vi "filterReadTimeout.vi"(8 "error in (no error)":errorcluster, 9 "matchChar":string, 10 "timeoutMs":u32=2000, 11 "filterPort":refnum<visa-resource-name>) -> (0 "error out":errorcluster, 2 "rxData":string, 3 "filterPortOut":refnum<visa-resource-name>)   [LabVIEW 2018]
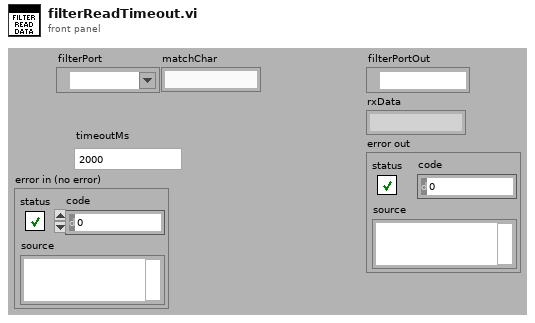
[diagram p1: front panel]
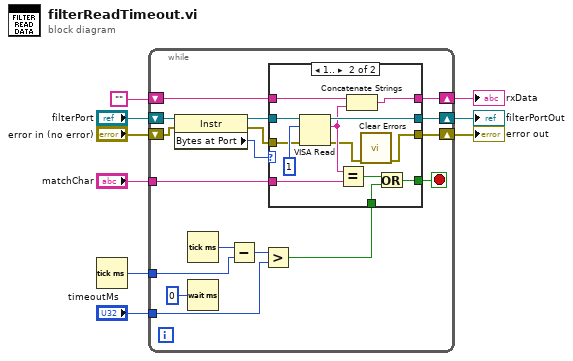
[diagram p0: block diagram]
diagram:
  n1 = Tick Count (ms)() -> (millisecond timer value=w8:u32)
  n2 = while {
    shift-left: "" -> [w25]
    shift-right: [w26] -> w4
    shift-right: [w23] -> w5
    shift-left: "filterPort" -> [w24]
    tunnel: w8 -> [w21]
    tunnel: "timeoutMs" -> [w18]
    shift-right: [w14] -> w2
    shift-left: "error in (no error)" -> [w15]
    tunnel: "matchChar" -> [w12]
    stop <- w11 stop-if-true
    n3 = property class="Instr"(reference=w24, error in=w15) -> (reference out=w17:refnum<visa-resource-name>, error out=w13:errorcluster, "Bytes at Port"=w16:u32)
    n4 = Tick Count (ms)() -> (millisecond timer value=w22:u32)
    n5 = Wait (ms)(milliseconds to wait=u32 0) -> ()  [unwired: 1 out]
    n6 = Subtract(x=w22, y=w21) -> (x-y=w20:u32)
    n7 = Greater?(x=w20, y=w18) -> (0:w10:bool)
    n8 = case shown="1.." w16 {
      tunnel: [w30 w43] -> w26
      tunnel: w25 -> [w30 w42]
      tunnel: [w29 w41] -> w23
      tunnel: w17 -> [w29 w39]
      tunnel: [w28 w31] -> w14
      tunnel: w13 -> [w28 w38]
      tunnel: w12 -> [_ w36]
      tunnel: [w27 w34] -> w11
      tunnel: w10 -> [w27 w33]
      frame 0, Default {
      }
      frame 1.. {
        n9 = VISA Read(VISA resource name=w39, byte count=u32 1, error in (no error)=w38) -> (VISA resource name out=w41:refnum<visa-resource-name>, read buffer=w37:string, error out=w32:errorcluster)  [unwired: 1 out]
        n10 = Equal?(x=w37, y=w36) -> (x = y?=w35:bool)
        n11 = Concatenate Strings(w42, w37) -> (w43:string)
        n12 = call <vilib>:"Clear Errors.vi"("error in (no error)"=w32) -> ("error out"=w31:errorcluster)  [unwired: 5 in, 1 out]
        n13 = Or(x=w35, y=w33) -> (x .or. y?=w34:bool)
      }
    }
  }
  "filterPortOut" <- w5
  "rxData" <- w4
  "error out" <- w2
